vi "Close.vi"(8 "error in (no error)":errorcluster, 11 "Data Grid in":refnum<class "Data Grid.lvclass">) -> (0 "error out":errorcluster, 3 "Data Grid out":refnum<class "Data Grid.lvclass">)   [LabVIEW 2013, in "Table Manager.lvlib" / "Data Grid.lvclass"]
uses:
  Data Grid.lvclass
  Table Manager/Table Manager.lvclass
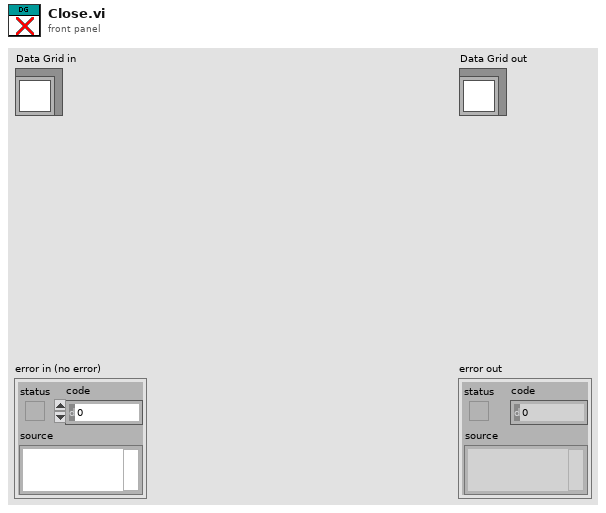
[diagram p1: front panel]
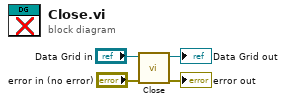
[diagram p0: block diagram]
diagram:
  n1 = call-parent "Close.vi"("error in (no error)"="error in (no error)", "table manager in"="Data Grid in") -> ("error out"=→"error out":errorcluster, "table manager out"=→"Data Grid out":refnum<class "Data Grid.lvclass">)  [unwired: 8 in]
